vi "Decompose Cluster - Mixed - Element Count.vi"() -> ()   [LabVIEW 2017, in "Composition.Tests.lvlib"]
uses:
  Composition.Tests.lvlib
  Composition/Composition.lvlib
  <vilib>/addons/_JKI Toolkits/Caraya/classes/Test/Test.lvclass
  <vilib>/addons/_JKI Toolkits/Caraya/classes/Assert/Assert.lvclass
panel:
  out "error out":errorcluster
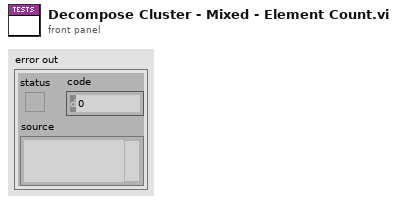
[diagram p1: front panel]
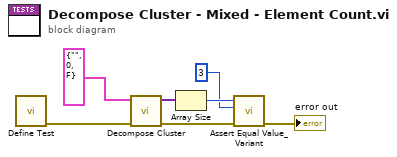
[diagram p0: block diagram]
diagram:
  n1 = call <vilib>:"Define Test.vi"() -> ("error out"=w4:errorcluster)  [unwired: 11 in]
  n2 = call "Decompose Cluster.vi"("error in (no error)"=w4, "Cluster"=cluster{string, i32, bool} {"", 0, FALSE}) -> ("error out"=w6:errorcluster, "Cluster Elements"=w3:variant[])  [unwired: 8 in]
  n3 = Array Size(array=w3) -> (size(s)=w2:i32)
  n4 = call <vilib>:"Assert Equal Value_Variant.vi"("error in (no error)"=w6, "Y"=3 ("Expected"), "X"=w2) -> ("error out"=→"error out":errorcluster)  [unwired: 8 in]
